vi "NATIONAL_INSTRUMENTS_TEMPLATE_model_info.vi"(11 "clear":bool) -> (0 "modelName":string, 1 "Outputs":T1[](array[typedef]), 2 "Inputs":T1[](array[typedef]), 3 "Parameters":T1[](array[typedef]), 4 "baseRate":dbl=0.01, 5 "Signals":T1[](array[typedef]))   [LabVIEW 2019]
uses:
  Program Files (x86)/National Instruments/LabVIEW 2019/project/NI VeriStand/LabVIEW Model Generator.llb/LV_SignalAttribute.ctl
panel:
  in  "Signals in":T1[](array[typedef])
  in  "Inputs in":T1[](array[typedef])
  in  "baseRate in":dbl
  in  "Outputs in":T1[](array[typedef])
  in  "modelName in":string="EPTxBasicExampleRT1.0"
  in  "Parameters in":T1[](array[typedef])
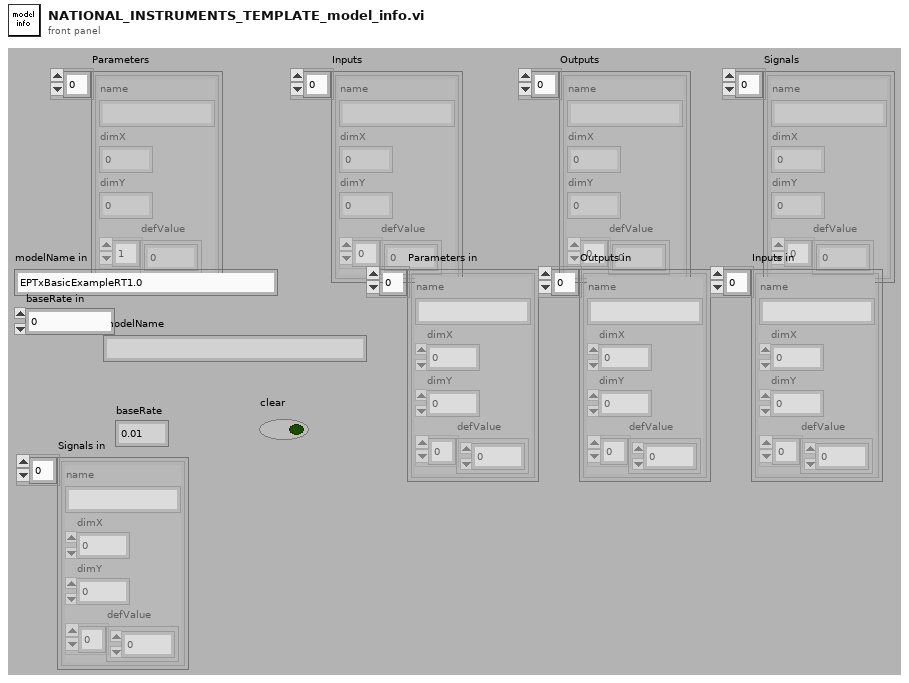
[diagram p1: front panel]
types:
  T1 = typedef "LV_SignalAttribute.ctl" = cluster{"name":string, "dimX":i32, "dimY":i32, "defValue":dbl[]}
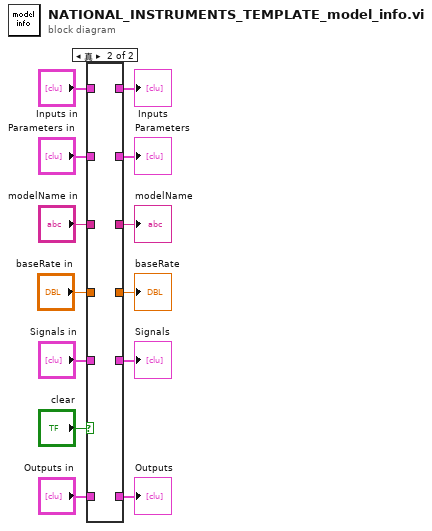
[diagram p0: block diagram]
diagram:
  n1 = case shown="真" "clear" {
    tunnel: "Parameters in" -> [w19 _]
    tunnel: [w19 _] -> w11
    tunnel: "modelName in" -> [w18 _]
    tunnel: [w18 _] -> w9
    tunnel: "Outputs in" -> [w17 _]
    tunnel: [w17 _] -> w7
    tunnel: "baseRate in" -> [w16 _]
    tunnel: [w16 _] -> w5
    tunnel: "Inputs in" -> [w15 _]
    tunnel: [w15 _] -> w3
    tunnel: [w14 _] -> w1
    tunnel: "Signals in" -> [w14 _]
    frame False {
    }
    frame True {
    }
  }
  "Parameters" <- w11
  "Inputs" <- w3
  "Outputs" <- w7
  "modelName" <- w9
  "baseRate" <- w5
  "Signals" <- w1
